vi "Dynamic Event basic.vi"() -> ()   [LabVIEW 2022 SP3]
panel:
  in  "String":string
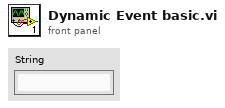
[diagram p1: front panel]
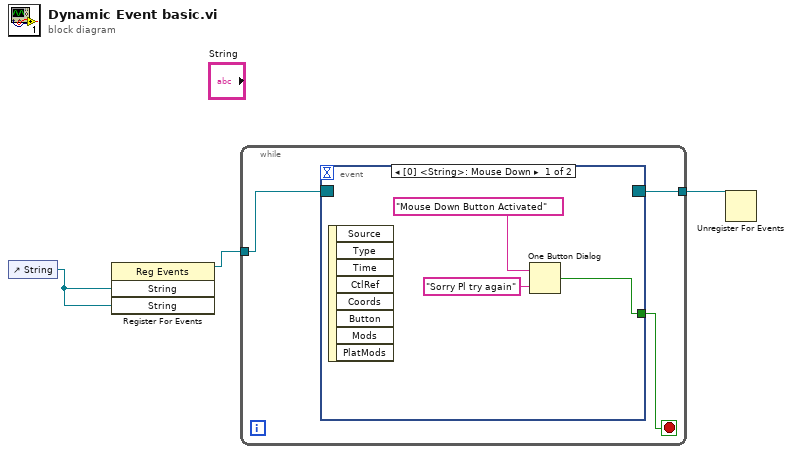
[diagram p0: block diagram]
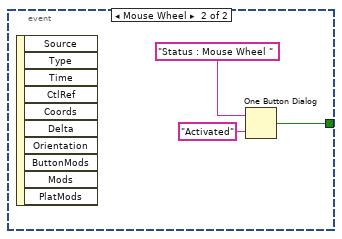
[diagram p2: hidden frame]
diagram:
  n1 = control-ref of="String"() -> (w3:refnum<vi>)
  n2 = register-events(w3, w3) -> (reference out=w2:refnum<event-registration>)  [unwired: 2 in, 1 out]
  n3 = while {
    tunnel: w2 -> [w6]
    tunnel: [w5] -> w1
    stop <- w4 stop-if-true
    n4 = event shown="[0] <String>: Mouse Down" {
      selector: w6 -> [_ _]
      dyn-events: [_ _] -> w5
      timeout: _ -> [_ _]
      tunnel: [w7 w10] -> w4
      event Mouse Down {
        n5 = event-data() -> ()  [unwired: 1 in, 8 out]
        n6 = One Button Dialog(message="Mouse Down Button Activated", button name ("OK")="Sorry Pl try again") -> (true=w7:bool)
      }
      event Mouse Wheel {
        n7 = event-data() -> ()  [unwired: 1 in, 10 out]
        n8 = One Button Dialog(message="Status : Mouse Wheel ", button name ("OK")="Activated") -> (true=w10:bool)
      }
    }
  }
  n9 = Unregister For Events(event registration refnum=w1) -> ()  [unwired: 1 in, 1 out]
